vi "Initialise Global variables.vi"(8 "error in (no error)":errorcluster, 11 "StageSPIM in":refnum<class "StageSPIM.lvclass">) -> (0 "error out":errorcluster, 3 "StageSPIM out":refnum<class "StageSPIM.lvclass">)   [LabVIEW 2012, in "StageSPIM.lvclass"]
uses:
  StageSPIM.lvclass
  PI drivers/Low Level/Communication.llb/Available interfaces.ctl
  PI drivers/Low Level/Communication.llb/Available DLLs.ctl
  StageSPIM.lvclass/StageSPIM.ctl
  PI drivers/Low Level/Communication.llb/Available DLL interfaces.ctl
  PI drivers/Low Level/Communication.llb/Global1.vi
  PI drivers/Low Level/Communication.llb/Global DaisyChain.vi
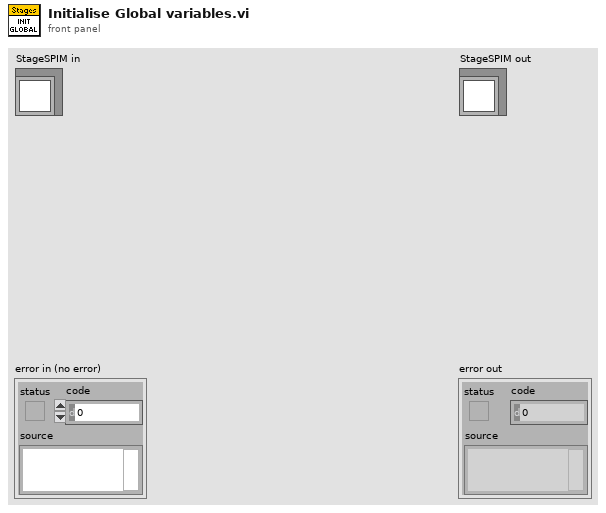
[diagram p1: front panel]
types:
  T1 = enum16{"C844_IsDLLAvailable", "C844_ConnectRS232", "C844_ConnectNIgpib", "C844_IsConnected", "C844_CloseConnection", "C844_GcsCommandset", "C844_GetError", "C844_GcsGetAnswerSize", "C844_GcsGetAnswer", "C843_IsDLLAvailable", "C843_Connect", "C843_IsConnected", "C843_CloseConnection", "C843_GcsCommandset", "C843_GetError", "C843_GcsGetAnswerSize", "C843_GcsGetAnswer", "E710_IsDLLAvailable", "E710_ConnectRS232", "E710_ConnectNIgpib", "E710_IsConnected", "E710_CloseConnection", "E710_GcsCommandset", "E710_GetError", "E710_GcsGetAnswerSize", "E710_GcsGetAnswer", "C843_PM_IsDLLAvailable", "C843_PM_Connect", "C843_PM_IsConnected", "C843_PM_CloseConnection", "C843_PM_GcsCommandset", "C843_PM_GetError", "C843_PM_GcsGetAnswerSize", "C843_PM_GcsGetAnswer", "C843_PM_GetCurrentBoardID", "C843_GetCurrentBoardID", "C865_IsDLLAvailable", "C865_ConnectRS232", "C865_IsConnected", "C865_CloseConnection", "C865_GcsCommandset", "C865_GetError", "C865_GcsGetAnswerSize", "C865_GcsGetAnswer", "C865_GetCurrentInterfaceID", "E761_ConnectPciBoard", "DefineSystem", "CloseConnection", "IsConnected", "ConnectRS232", "ConnectNIgpib", "ConnectPciBoard", "ConnectTCPIP", "GetError", "GcsCommandset", "GCSGetAnswerSize", "GcsGetAnswer"}
  T2 = enum16{"C844_IsDLLAvailable", "C844_ConnectRS232", "C844_ConnectNIgpib", "C844_IsConnected", "C844_CloseConnection", "C844_GcsCommandset", "C844_GetError", "C844_GcsGetAnswerSize", "C844_GcsGetAnswer", "C843_IsDLLAvailable", "C843_Connect", "C843_IsConnected", "C843_CloseConnection", "C843_GcsCommandset", "C843_GetError", "C843_GcsGetAnswerSize", "C843_GcsGetAnswer", "E710_IsDLLAvailable", "E710_ConnectRS232", "E710_ConnectNIgpib", "E710_IsConnected", "E710_CloseConnection", "E710_GcsCommandset", "E710_GetError", "E710_GcsGetAnswerSize", "E710_GcsGetAnswer", "C843_PM_IsDLLAvailable", "C843_PM_Connect", "C843_PM_IsConnected", "C843_PM_CloseConnection", "C843_PM_GcsCommandset", "C843_PM_GetError", "C843_PM_GcsGetAnswerSize", "C843_PM_GcsGetAnswer", "C843_PM_GetCurrentBoardID", "C843_GetCurrentBoardID", "C865_IsDLLAvailable", "C865_ConnectRS232", "C865_IsConnected", "C865_CloseConnection", "C865_GcsCommandset", "C865_GetError", "C865_GcsGetAnswerSize", "C865_GcsGetAnswer", "C865_GetCurrentInterfaceID", "E761_ConnectPciBoard", "DefineSystem", "CloseConnection", "IsConnected", "ConnectRS232", "ConnectNIgpib", "ConnectPciBoard", "ConnectTCPIP", "GetError", "GcsCommandset", "GCSGetAnswerSize", "GcsGetAnswer", "CloseDaisyChain", "OpenRS232DaisyChain", "ConnectDaisyChainDevice", "ConnectUSB", "ListUSB", "OpenUSBDaisyChain"}
  T3 = enum16{"C844_IsDLLAvailable", "C844_ConnectRS232", "C844_ConnectNIgpib", "C844_IsConnected", "C844_CloseConnection", "C844_GcsCommandset", "C844_GetError", "C844_GcsGetAnswerSize", "C844_GcsGetAnswer", "C843_IsDLLAvailable", "C843_Connect", "C843_IsConnected", "C843_CloseConnection", "C843_GcsCommandset", "C843_GetError", "C843_GcsGetAnswerSize", "C843_GcsGetAnswer", "E710_IsDLLAvailable", "E710_ConnectRS232", "E710_ConnectNIgpib", "E710_IsConnected", "E710_CloseConnection", "E710_GcsCommandset", "E710_GetError", "E710_GcsGetAnswerSize", "E710_GcsGetAnswer", "C843_PM_IsDLLAvailable", "C843_PM_Connect", "C843_PM_IsConnected", "C843_PM_CloseConnection", "C843_PM_GcsCommandset", "C843_PM_GetError", "C843_PM_GcsGetAnswerSize", "C843_PM_GcsGetAnswer", "C843_PM_GetCurrentBoardID", "C843_GetCurrentBoardID", "C865_IsDLLAvailable", "C865_ConnectRS232", "C865_IsConnected", "C865_CloseConnection", "C865_GcsCommandset", "C865_GetError", "C865_GcsGetAnswerSize", "C865_GcsGetAnswer", "C865_GetCurrentInterfaceID", "E761_ConnectPciBoard", "DefineSystem", "CloseConnection", "IsConnected", "ConnectRS232", "ConnectNIgpib", "ConnectPciBoard", "ConnectTCPIP", "GetError", "GcsCommandset", "GCSGetAnswerSize", "GcsGetAnswer", "CloseDaisyChain", "OpenRS232DaisyChain", "ConnectDaisyChainDevice"}
  T4 = typedef "Available DLLs.ctl" = u16
  T5 = typedef "Available interfaces.ctl" = u16
  T6 = typedef "StageSPIM.lvclass/port_control.ctl" = i32
  T7 = typedef "StageSPIM.lvclass/baud_rate_control.ctl" = u16
  T8 = typedef "StageSPIM.lvclass/connection_type.ctl" = enum16{"RS232", "RS232 DaisyChain", "USB", "USB_DaisyChain"}
  T9 = typedef "Available DLL interfaces.ctl" = u16
  T10 = cluster{"DLL for Device":T4, "DLL Interface":T9, "Parameter":string}[]
  T11 = cluster{"RS232 Portnumber":i32, "Timeout":i32, "RS232 Baud rate":u32, "Interface":T5, "GPIB Bus":i32, "GPIB Address":i32, "GPIB Mode":i32}[]
  T12 = cluster{"input XON/XOFF":bool, "input HW Handshake":bool, "input alt HW HShk":bool, "output XON/XOFF":bool, "output HW Handshake":bool, "output alt HW HShk":bool, "XOFF byte ":u8, "XON byte":u8, "parity error byte":u16}[]
  T13 = cluster{"RS232 Portnumber":i32, "Timeout":i32, "RS232 Baud rate":u32, "Interface":T5, "GPIB Bus":i32, "GPIB Address":i32, "GPIB Mode":i32}
  T14 = cluster{"DLL for Device":T4, "DLL Interface":T9, "Parameter":string}
  T15 = cluster{"input XON/XOFF":bool, "input HW Handshake":bool, "input alt HW HShk":bool, "output XON/XOFF":bool, "output HW Handshake":bool, "output alt HW HShk":bool, "XOFF byte ":u8, "XON byte":u8, "parity error byte":u16}
  T16 = cluster{"No. of devices":i32, "Port ID":i32, "Devices":string[], "Description":string}[]
  T17 = cluster{"No. of devices":i32, "Port ID":i32, "Devices":string[], "Description":string}
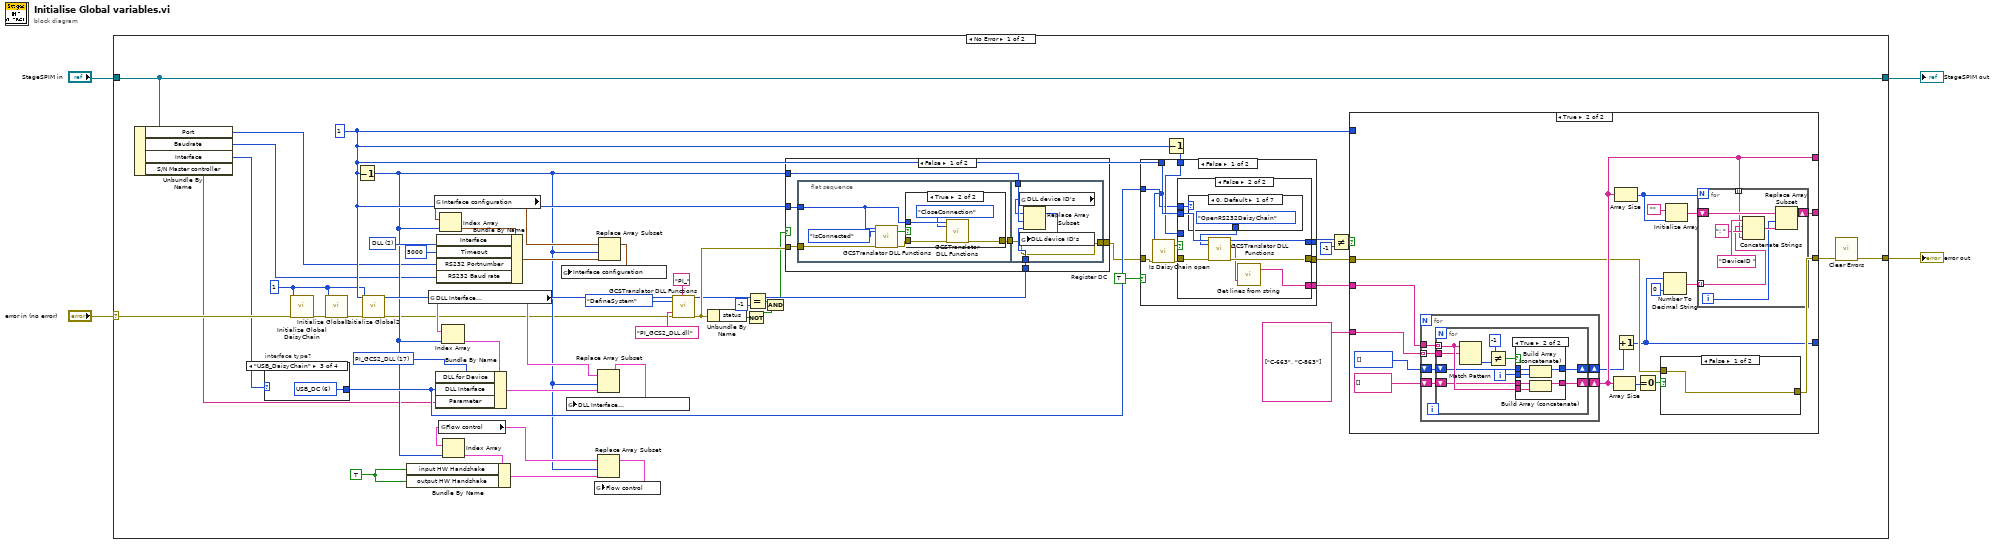
[diagram p0: block diagram]
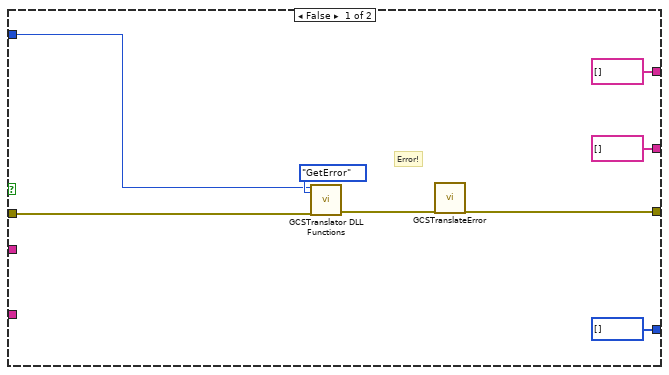
[diagram p2: hidden frame]
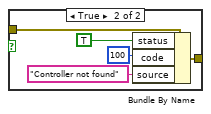
[diagram p4: hidden frame]
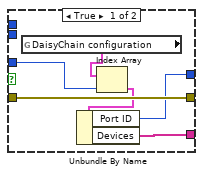
[diagram p5: hidden frame]
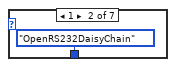
[diagram p6: hidden frame]
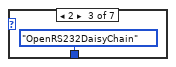
[diagram p7: hidden frame]
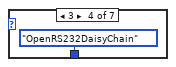
[diagram p8: hidden frame]
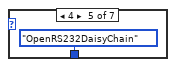
[diagram p9: hidden frame]
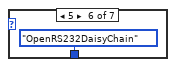
[diagram p10: hidden frame]
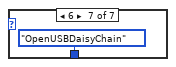
[diagram p11: hidden frame]
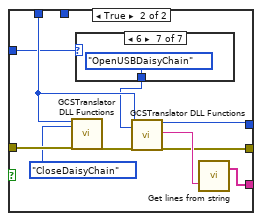
[diagram p12: hidden frame]
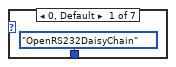
[diagram p13: hidden frame]
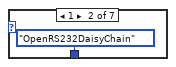
[diagram p14: hidden frame]
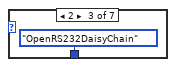
[diagram p15: hidden frame]
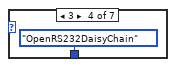
[diagram p16: hidden frame]
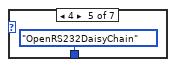
[diagram p17: hidden frame]
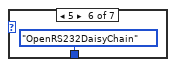
[diagram p18: hidden frame]
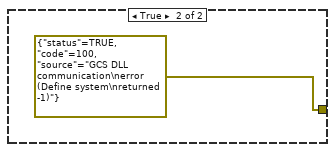
[diagram p20: hidden frame]
diagram:
  n1 = case shown="No Error" "error in (no error)" {
    selector: "error in (no error)" -> [w11 w193]
    tunnel: [w5 w193] -> w3
    tunnel: [w10 w192] -> w1
    tunnel: "StageSPIM in" -> [w10 w192]
    frame No Error {
      w13 = 1 ("System no.")
      w31 = T4 17 items=["C-843", "C-844", "E-710", "C-843.PM", "C-865", "E-761", "Mercury", "E-755", "E-753", "C-866", "E-712", "E-725", "E-861", "C-867", "E-517", "E-816", "E-709", "PI_GCS2_DLL"] ("DLL for Device")
      w48 = T5 2 items=["RS232", "GPIB", "DLL", "TCP-IP"] ("Interface")
      w46 = TRUE ("Bundle Element")
      w53 = 1 ("System no.")
      w54 = TRUE  # Register DC
      n2 = Unbundle By Name(w10) -> ("Port"=w7:T6, "Baudrate"=w6:T7, "Interface"=w8:T8, "S/N Master controller"=w9:string)
      n3 = case "interface type?" shown="\"USB_DaisyChain\"" w8 {
        tunnel: [w188 w189 w190 w191] -> w52
        frame "RS232", Default {
          w188 = T9 0 items=["RS232", "GPIB", "Board", "TCP-IP", "USB", "RS232_DC", "USB_DC"] ("DLL Interface")
        }
        frame "USB" {
          w189 = T9 4 items=["RS232", "GPIB", "Board", "TCP-IP", "USB", "RS232_DC", "USB_DC"] ("DLL Interface")
        }
        frame "USB_DaisyChain" {
          w190 = T9 6 items=["RS232", "GPIB", "Board", "TCP-IP", "USB", "RS232_DC", "USB_DC"] ("DLL Interface")
        }
        frame "RS232 DaisyChain" {
          w191 = T9 5 items=["RS232", "GPIB", "Board", "TCP-IP", "USB", "RS232_DC", "USB_DC"] ("DLL Interface")
        }
      }
      n4 = call "Initialize Global DaisyChain.vi"("System no."=w13, "error in"=w11) -> ("error out"=w15:errorcluster)  [unwired: 17 in]
      n5 = call "Initialize Global1.vi"("System no."=w13, "error in"=w15) -> ("error out"=w14:errorcluster)  [unwired: 17 in]
      n6 = Decrement(x=w53) -> (x-1=w26:i32)
      n7 = call "Initialize Global2.vi"("System no."=w13, "error in"=w14) -> ("error out"=w12:errorcluster)  [unwired: 17 in]
      n8 = global read "Global1.vi" "DLL Interface\nConfiguration"() -> (w37:T10)
      n9 = global read "Global1.vi" "Interface configuration"() -> (w38:T11)
      n10 = global read "Global1.vi" "Flow control"() -> (w36:T12)
      n11 = Index Array(array=w38, index=w26) -> (element=w49:T13)
      n12 = Bundle By Name(cluster=w49, "Interface"=w48, "Timeout"=5000, "RS232 Portnumber"=w7, "RS232 Baud rate"=w6) -> (w41:T13)
      n13 = Index Array(array=w37, index=w26) -> (element=w45:T14)
      n14 = Bundle By Name(cluster=w45, "DLL for Device"=w31, "DLL Interface"=w52, "Parameter"=w9) -> (w40:T14)
      n15 = Index Array(array=w36, index=w26) -> (element=w47:T15)
      n16 = Bundle By Name(cluster=w47, "input HW Handshake"=w46, "output HW Handshake"=w46) -> (w39:T15)
      n17 = Replace Array Subset(array=w37, new element=w40, index=w26) -> (w43:T10)
      n18 = global write "Global1.vi" "DLL Interface\nConfiguration"(w43) -> ()
      n19 = Replace Array Subset(array=w36, new element=w39, index=w26) -> (w44:T12)
      n20 = global write "Global1.vi" "Flow control"(w44) -> ()
      n21 = Replace Array Subset(array=w38, new element=w41, index=w26) -> (w42:T11)
      n22 = global write "Global1.vi" "Interface configuration"(w42) -> ()
      n23 = call "GCSTranslator DLL Functions.vi"("System no."=w53, "Function"=T1."DefineSystem", "String input"="PI_GCS2_DLL.dll", "error in"=w12, "String input 2"="PI_") -> ("DLL I32 Return value"=w25:i32, "error out"=w27:errorcluster)  [unwired: 10 in, 3 out]
      n24 = Unbundle By Name(w27) -> ("status"=w29:bool)
      n25 = Not(x=w29) -> (.not. x?=w28:bool)
      n26 = Equal?(x=w25, y=-1) -> (x = y?=w30:bool)
      n27 = And(x=w30, y=w28) -> (x .and. y?=w24:bool)
      n28 = case shown="False" w24 {
        tunnel: w53 -> [w165 _]
        tunnel: w27 -> [w168 _]
        tunnel: w26 -> [w170 _]
        tunnel: w25 -> [w169 _]
        tunnel: [w166 errorcluster {"status"=TRUE, "code"=100, "source"="GCS DLL communication\nerror (Define system\nreturned -1)"} ("error out")] -> w51
        frame False {
          n29 = flat-sequence {
            tunnel: w168 -> [w173]
            tunnel: [w172] -> w167
            tunnel: w165 -> [w171]
            tunnel: w170 -> [w186]
            tunnel: w169 -> [w183]
            tunnel: w167 -> [w182]
            tunnel: [w182] -> w166
            frame #0 {
              n30 = call "GCSTranslator DLL Functions.vi"("System no."=w171, "Function"=T1."IsConnected", "error in"=w173) -> ("Boolean output"=w176:bool, "error out"=w175:errorcluster)  [unwired: 12 in, 3 out]
              n31 = case shown="True" w176 {
                tunnel: w171 -> [_ w181]
                tunnel: w175 -> [w177 w180]
                tunnel: [w177 w179] -> w172
                frame False {
                }
                frame True {
                  n32 = call "GCSTranslator DLL Functions.vi"("System no."=w181, "Function"=T1."CloseConnection", "error in"=w180) -> ("error out"=w179:errorcluster)  [unwired: 12 in, 4 out]
                }
              }
            }
            frame #1 {
              n33 = global read "Global1.vi" "DLL device ID's"() -> (w184:i32[])
              n34 = Replace Array Subset(array=w184, new element=w183, index=w186) -> (w185:i32[])
              n35 = global write "Global1.vi" "DLL device ID's"(w185) -> ()
            }
          }
        }
        frame True {
        }
      }
      n36 = Decrement(x=w53) -> (x-1=w22:i32)
      n37 = case shown="False" w54 {
        tunnel: w51 -> [w126 w157]
        tunnel: [w122 w148] -> w18
        tunnel: w53 -> [w124 w154]
        tunnel: [w121 w151] -> w20
        tunnel: w22 -> [w120 _]
        tunnel: [w119 w152] -> w21
        tunnel: w52 -> [w118 w150]
        frame False {
          n38 = call "Is DaisyChain open.vi"("System no."=w124, "error in"=w126) -> ("DC open?"=w125:bool, "error out"=w123:errorcluster)  [unwired: 15 in, 1 out]
          n39 = case shown="False" w125 {
            tunnel: w124 -> [_ w140]
            tunnel: w123 -> [w132 w139]
            tunnel: [w132 w138] -> w122
            tunnel: [w129 w137] -> w121
            tunnel: w120 -> [w128 _]
            tunnel: [w127 w135] -> w119
            tunnel: w118 -> [_ w133]
            frame True {
              n40 = global read "Global DaisyChain.vi" "DaisyChain configuration"() -> (w130:T16)
              n41 = Index Array(array=w130, index=w128) -> (element=w131:T17)
              n42 = Unbundle By Name(w131) -> ("Port ID"=w129:i32, "Devices"=w127:string[])
            }
            frame False {
              n43 = case shown="0, Default" w133 {
                tunnel: [T2."OpenRS232DaisyChain" ("Function") T2."OpenRS232DaisyChain" ("Function") T2."OpenRS232DaisyChain" ("Function") T2."OpenRS232DaisyChain" ("Function") T2."OpenRS232DaisyChain" ("Function") T2."OpenRS232DaisyChain" ("Function") T2."OpenUSBDaisyChain" ("Function")] -> w134
                frame 0, Default {
                }
                frame 1 {
                }
                frame 2 {
                }
                frame 3 {
                }
                frame 4 {
                }
                frame 5 {
                }
                frame 6 {
                }
              }
              n44 = call "GCSTranslator DLL Functions.vi"("System no."=w140, "Function"=w134, "error in"=w139) -> ("DLL I32 Return value"=w137:i32, "String output"=w136:string, "error out"=w138:errorcluster)  [unwired: 12 in, 2 out]
              n45 = call "Get lines from string.vi"("Input string"=w136) -> ("Strings"=w135:string[])  [unwired: 17 in, 1 out]
            }
          }
        }
        frame True {
          n46 = call "GCSTranslator DLL Functions.vi"("System no."=w154, "Function"=T3."CloseDaisyChain", "error in"=w157) -> ("error out"=w155:errorcluster)  [unwired: 12 in, 4 out]
          n47 = case shown="6" w150 {
            tunnel: [T2."OpenRS232DaisyChain" ("Function") T2."OpenRS232DaisyChain" ("Function") T2."OpenRS232DaisyChain" ("Function") T2."OpenRS232DaisyChain" ("Function") T2."OpenRS232DaisyChain" ("Function") T2."OpenRS232DaisyChain" ("Function") T2."OpenUSBDaisyChain" ("Function")] -> w149
            frame 0, Default {
            }
            frame 1 {
            }
            frame 2 {
            }
            frame 3 {
            }
            frame 4 {
            }
            frame 5 {
            }
            frame 6 {
            }
          }
          n48 = call "GCSTranslator DLL Functions.vi"("System no."=w154, "Function"=w149, "error in"=w155) -> ("DLL I32 Return value"=w151:i32, "String output"=w153:string, "error out"=w148:errorcluster)  [unwired: 12 in, 2 out]
          n49 = call "Get lines from string.vi"("Input string"=w153) -> ("Strings"=w152:string[])  [unwired: 17 in, 1 out]
        }
      }
      n50 = Not Equal?(x=w20, y=-1) -> (x != y?=w17:bool)
      n51 = case shown="True" w17 {
        tunnel: [string[] [] w77] -> _
        tunnel: string[] ["C-663", "C-863"] -> [_ w72]
        tunnel: [w56 w71] -> w50
        tunnel: [string[] [] w70] -> _
        tunnel: w18 -> [w61 w69]
        tunnel: w21 -> [_ w68]
        tunnel: w53 -> [w60 _]
        tunnel: [i32[] [] w63] -> _
        frame False {
          # "Error!"
          n52 = call "GCSTranslator DLL Functions.vi"("System no."=w60, "Function"=T1."GetError", "error in"=w61) -> ("error out"=w57:errorcluster)  [unwired: 12 in, 4 out]
          n53 = call "GCSTranslateError.vi"("error in"=w57) -> ("error out"=w56:errorcluster)  [unwired: 16 in, 2 out]
        }
        frame True {
          n54 = for {
            tunnel: w72 -> [w84] mode=indexing
            tunnel: w68 -> [w82]
            shift-right: [w83] -> w70
            shift-left: string[] [] -> [w85]
            shift-right: [w80] -> w64
            shift-left: i32[] [] -> [w81]
            n55 = for {
              tunnel: w82 -> [w93] mode=indexing
              shift-right: [w92] -> w83
              shift-left: w85 -> [w91]
              tunnel: w84 -> [w90]
              shift-right: [w89] -> w80
              shift-left: w81 -> [w88]
              i -> [w86]
              n56 = Match Pattern(string=w93, regular expression=w90) -> (offset past match=w87:i32)  [unwired: 1 in, 3 out]
              n57 = Not Equal?(x=-1 ("y"), y=w87) -> (x != y?=w94:bool)
              n58 = case shown="True" w94 {
                tunnel: w93 -> [_ w102]
                tunnel: [w97 w103] -> w92
                tunnel: w91 -> [w97 w101]
                tunnel: [w96 w100] -> w89
                tunnel: w88 -> [w96 w99]
                tunnel: w86 -> [_ w98]
                frame False {
                }
                frame True {
                  n59 = Build Array (concatenate)(w99, w98) -> (w100:i32[])
                  n60 = Build Array (concatenate)(w101, w102) -> (w103:string[])
                }
              }
            }
          }
          n61 = Array Size(array=w70) -> (size(s)=w74:i32)
          n62 = Array Size(array=w70) -> (size(s)=w76:i32)
          n63 = Increment(x=w64) -> (x+1=w63:i32[])
          n64 = Equal To 0?(x=w74) -> (x = 0?=w73:bool)
          n65 = case shown="False" w73 {
            tunnel: [w104 w106] -> w71
            tunnel: w69 -> [w104 w105]
            frame False {
            }
            frame True {
              n66 = Bundle By Name(cluster=w105, "status"=TRUE, "code"=100 ("Bundle Element"), "source"="Controller not found" ("Bundle Element")) -> (w106:errorcluster)
            }
          }
          n67 = Number To Decimal String(number=w63, width (-)=i16 0) -> (decimal integer string=w65:string[])
          n68 = Initialize Array("", w76) -> (w79:string[])
          n69 = for {
            N: w76 -> [_]
            shift-right: [w115] -> w77
            shift-left: w79 -> [w117]
            tunnel: w70 -> [w111] mode=indexing
            tunnel: w65 -> [w110] mode=indexing
            i -> [w113]
            n70 = Concatenate Strings("DeviceID ", w110, ": " ("string"), w111) -> (w116:string)
            n71 = Replace Array Subset(array=w117, new element=w116, index=w113) -> (w115:string[])
          }
        }
      }
      n72 = call <vilib>:"Clear Errors.vi"("error in (no error)"=w50) -> ("error out"=w5:errorcluster)  [unwired: 6 in]
    }
    frame Error {
    }
  }
  "error out" <- w3
  "StageSPIM out" <- w1
